vi "Write Test Stand Class.vi"(8 "error in (no error)":errorcluster, 10 "Generic Test Stand.lvclass":refnum<class "Generic Test Stand.lvclass">, 11 "Init UI Process in":refnum<class "Init UI Process.lvclass">) -> (0 "error out":errorcluster, 3 "Init UI Process out":refnum<class "Init UI Process.lvclass">)   [LabVIEW 2019, in "User Interface Process.lvlib" / "Init UI Process.lvclass"]
uses:
  Init UI Process.lvclass
  Generic Test Stand/Generic Test Stand.lvclass
  Init UI Process.lvclass/Init UI Process.ctl
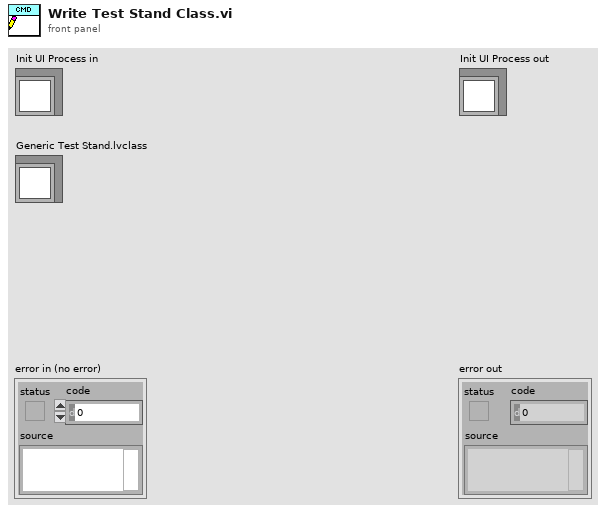
[diagram p1: front panel]
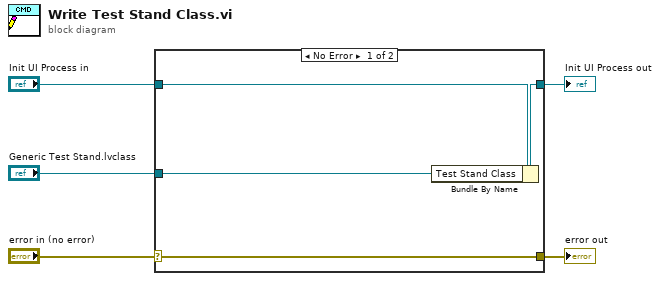
[diagram p0: block diagram]
diagram:
  n1 = case shown="No Error" "error in (no error)" {
    selector: "error in (no error)" -> [w9 w10]
    tunnel: [w9 w10] -> w4
    tunnel: [w7 w11] -> w2
    tunnel: "Init UI Process in" -> [w8 w11]
    tunnel: "Generic Test Stand.lvclass" -> [w6 _]
    frame No Error {
      n2 = Bundle By Name(cluster=w8, "Test Stand Class"=w6) -> (w7:refnum<class "Init UI Process.lvclass">)
    }
    frame Error {
    }
  }
  "error out" <- w4
  "Init UI Process out" <- w2
